vi "Recurse.vi"(6 "Teller":refnum<class "Teller.lvclass">, 7 "Actor in":refnum<class "Actor.lvclass">) -> (0 "Error out":errorcluster, 5 "Actor out":refnum<class "Actor.lvclass">)   [LabVIEW 2025, in "_Template.lvlib" / "Templates.lvlib" / "TEMPLATE jettl Msg.lvlib"]
uses:
  TEMPLATE jettl Msg.lvlib
  jettl/jettl/jettl.lvlib
  TEMPLATE Msg Output/TEMPLATE Msg Output.lvlib
  Init Msg.vi
  jettl/jettl/Actor/Actor.lvclass
  jettl/jettl/Teller/Teller.lvclass
panel:
  # "This front panel should not be manipulated."
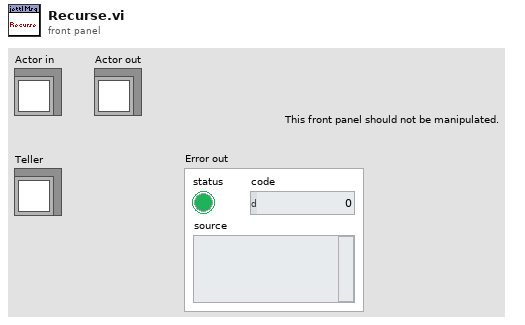
[diagram p1: front panel]
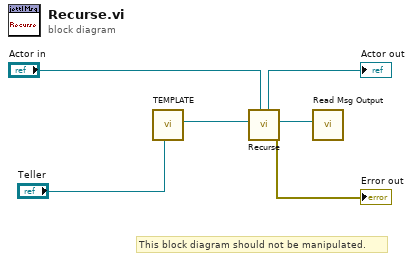
[diagram p0: block diagram]
diagram:
  # "This block diagram should not be manipulated."
  n1 = call-poly "TEMPLATE.vi"("Teller"="Teller") -> ("Msg"=w2:refnum<class "Msg.lvclass">)  [unwired: 10 in]
  n2 = call "Recurse.vi"("Actor in"="Actor in", "Msg"=w2) -> ("Error out"=→"Error out":errorcluster, "Msg Output"=w3:refnum<class "Msg Output.lvclass">, "Actor out"=→"Actor out":refnum<class "Actor.lvclass">)  [unwired: 7 in]
  n3 = call "Read Msg Output.vi"("Msg Output"=w3) -> ()  [unwired: 10 in, 1 out]
